vi "Pcre2SetCharacterTables8.vi"(8 "error in":errorcluster, 10 "pTable":u64 format="%.0x", 11 "pCompileContext":u64 format="%.0x") -> (0 "error out":errorcluster, 3 "pCompileContext":u64 format="%.0x")   [LabVIEW 2021, in "libpcre2-8.lvlib"]
uses:
  libpcre2-8.lvlib
  libpcre2-8-x32.dll
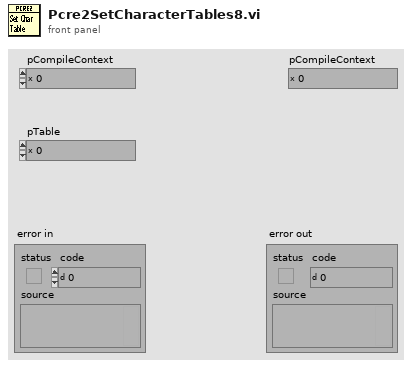
[diagram p1: front panel]
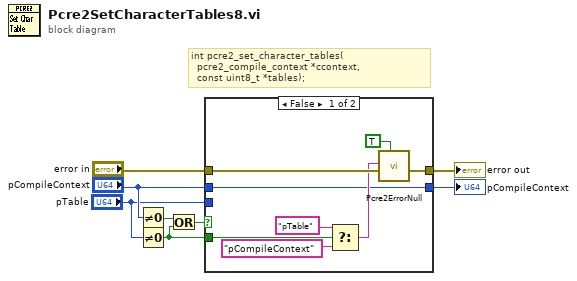
[diagram p0: block diagram]
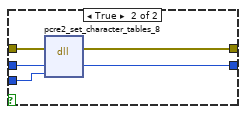
[diagram p2: hidden frame]
diagram:
  # "int pcre2_set_character_tables(\n  pcre2_compile_context *ccontext,\n  const uint8_t *tables);"
  n1 = Not Equal To 0?(x="pCompileContext") -> (x != 0?=w3:bool)
  n2 = Not Equal To 0?(x="pTable") -> (x != 0?=w1:bool)
  n3 = Or(x=w3, y=w1) -> (x .or. y?=w2:bool)
  n4 = case shown="False" w2 {
    tunnel: "error in" -> [w15 w21]
    tunnel: [w16 w20] -> w7
    tunnel: "pTable" -> [_ w19]
    tunnel: "pCompileContext" -> [w9 w18]
    tunnel: [w9 w17] -> w6
    tunnel: w1 -> [w13 _]
    frame False {
      n5 = Select(t="pTable", s=w13, f="pCompileContext") -> (s? t:f=w12:string)
      n6 = call "Pcre2ErrorNull.vi"("IsPointer? (F)"=TRUE, "error in"=w15, "What"=w12) -> ("error out"=w16:errorcluster)  [unwired: 8 in]
    }
    frame True {
      n7 = dll-call lib="libpcre2-8-x*.dll" fn="pcre2_set_character_tables_8"(error in=w21, "ccontext"=w18, "pTable"=w19) -> (error out=w20:errorcluster, "ccontext"=w17:u64)  [unwired: 4 in, 1 out]
    }
  }
  "error out" <- w7
  "pCompileContext" <- w6
